vi "ExSubCollectDisplayAdv.vi"(0 "Handle Cluster":T1, 1 "Display Title":string, 2 "Store flag":i8, 3 "error in (no error)":errorcluster, 4 "advanced display handle":refnum<k7>) -> (5 "Handle Cluster Out":T1, 6 "got frame":u32, 7 "error out":errorcluster)   [LabVIEW 2010]
panel:
  # "ExSubCollectDisplayStore:\nThis sub-VI checks to see if data has arrived from camera,  if so it then puts it in image object and displays it. If store switch is set it will also store it."
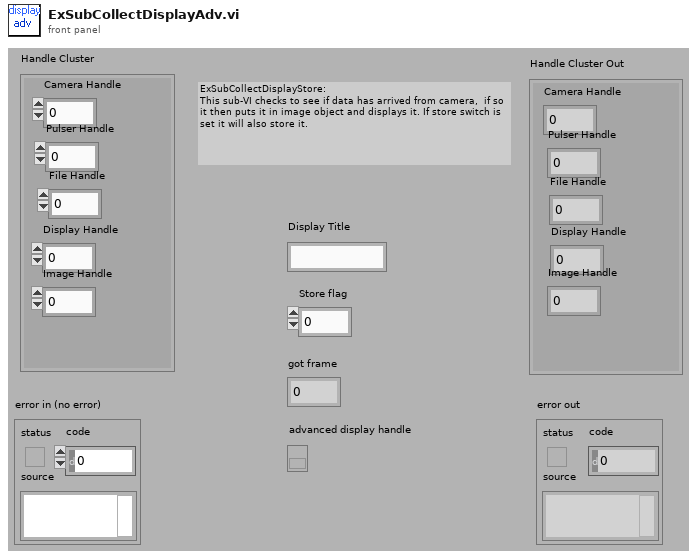
[diagram p1: front panel]
types:
  T1 = cluster{"Camera Handle":u32, "Pulser Handle":u32, "File Handle":u32, "Display Handle":u32, "Image Handle":u32}
  T2 = cluster{"Camera Handle":u32, "Pulser Handle":u32, "File Handle":u32, "Display Handle":u32, "Data Handle":u32}
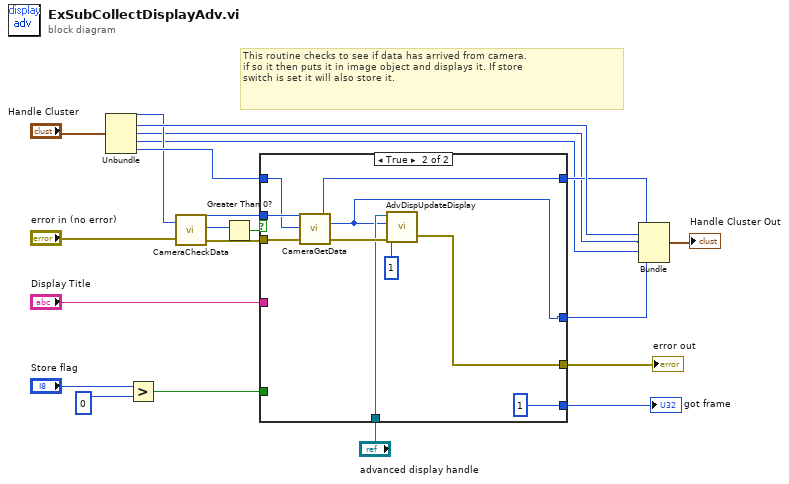
[diagram p0: block diagram]
diagram:
  # "This routine checks to see if data has arrived from camera.\nif so it then puts it in image object and displays it. If store \nswitch is set it will also store it."
  n1 = Unbundle("Handle Cluster") -> ("Camera Handle"=w10:u32, "Pulser Handle"=w13:u32, "File Handle"=w3:u32, "Display Handle"=w2:u32, "Image Handle"=w15:u32)
  n2 = Greater?(x="Store flag", y=0) -> (0:w6:bool)
  n3 = call <userlib>:"CameraCheckData.vi"("Camera Handle"=w10, "error in"="error in (no error)") -> ("Camera Handle"=w19:u32, "Number Of Frames Available"=w18:i32, "error out"=w17:errorcluster)
  n4 = Greater Than 0?(x=w18) -> (x > 0?=w20:bool)
  n5 = case shown="True" w20 {
    tunnel: w19 -> [w25 w35]
    tunnel: w17 -> [w24 w34]
    tunnel: w15 -> [w23 w32]
    tunnel: [w25 w33] -> w11
    tunnel: "Display Title" -> [_ _]
    tunnel: [w24 w29] -> w12
    tunnel: [w23 w26] -> w9
    tunnel: w6 -> [_ _]
    tunnel: [0 1] -> w5
    tunnel: "advanced display handle" -> [_ w28]
    frame False {
    }
    frame True {
      n6 = call <userlib>:"CameraGetData.vi"("error in"=w34, "Data Handle"=w32, "Camera Handle"=w35) -> ("error out"=w30:errorcluster, "Data Handle"=w26:u32, "Camera Handle"=w33:u32)
      n7 = call <userlib>:"AdvDispUpdateDisplay.vi"("error in (no error)"=w30, "Frame Number To Display"=1, "Image Handle"=w26, "SITKFULLDISPLAYLib.SITKFullDisplay"=w28) -> ("error out"=w29:errorcluster)  [unwired: 1 out]
    }
  }
  "error out" <- w12
  "got frame" <- w5
  n8 = Bundle("Camera Handle"=w11, "Pulser Handle"=w13, "File Handle"=w3, "Display Handle"=w2, "Data Handle"=w9) -> (→"Handle Cluster Out":T2)  [unwired: 1 in]
